vi "IsEnumArrayControl.vi"(8 "error in)":errorcluster, 11 "control reference in":refnum<vi>) -> (0 "error out":errorcluster, 1 "is enum array control":bool, 2 "array reference out":refnum<vi>, 3 "control reference out":refnum<vi>)   [LabVIEW 2020, in "MeasurementLink Measurement Server.lvlib"]
uses:
  MeasurementLink Measurement Server.lvlib
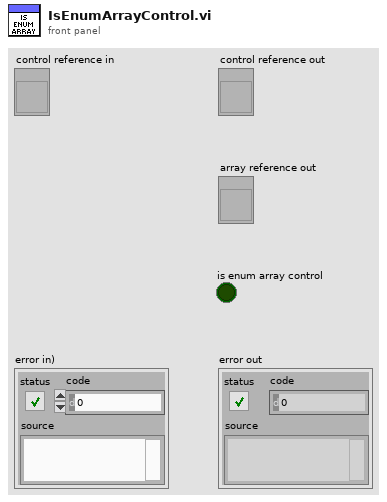
[diagram p1: front panel]
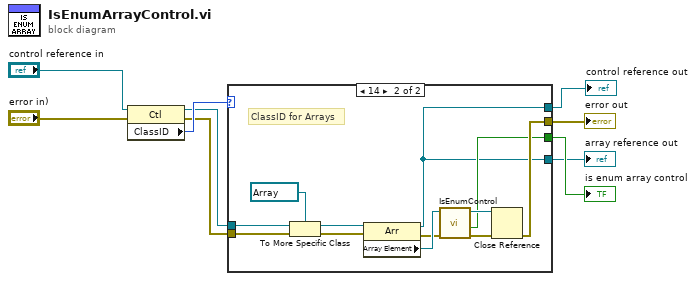
[diagram p0: block diagram]
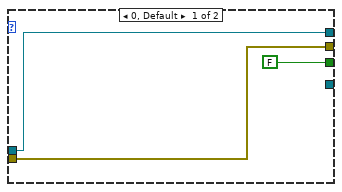
[diagram p2: hidden frame]
diagram:
  n1 = property class="Ctl"(reference="control reference in", error in="error in)") -> (reference out=w5:refnum<vi>, error out=w4:errorcluster, "ClassID"=w9:u32)
  n2 = case shown="14" w9 {
    tunnel: [FALSE w15] -> w6
    tunnel: w5 -> [w11 w23]
    tunnel: w4 -> [w10 w22]
    tunnel: [w11 w13] -> w2
    tunnel: [w10 w17] -> w3
    tunnel: [_ w13] -> w1
    frame 0, Default {
    }
    frame 14 {
      # "ClassID for Arrays"
      n3 = To More Specific Class(target class=refnum<vi> refnum ("Enum reference in"), reference=w23, error in=w22) -> (specific class reference=w14:refnum<vi>, error out=w21:errorcluster)
      n4 = property class="Arr"(reference=w14, error in=w21) -> (reference out=w13:refnum<vi>, error out=w16:errorcluster, "Array Element"=w20:refnum<vi>)
      n5 = call "IsEnumControl.vi"("error in (no error)"=w16, "Control reference in"=w20) -> ("error out"=w19:errorcluster, "IsEnumControl"=w15:bool, "Control reference out"=w18:refnum<vi>)  [unwired: 6 in, 1 out]
      n6 = Close Reference(reference=w18, error in (no error)=w19) -> (error out=w17:errorcluster)
    }
  }
  "control reference out" <- w2
  "is enum array control" <- w6
  "error out" <- w3
  "array reference out" <- w1
